vi "Read.vi"(2 "Que name":string, 5 "error in":errorcluster, 7 "Timeout (default 2s)":i32=2000) -> (4 "Message out":string, 6 "error out":errorcluster, 8 "Data":variant)   [LabVIEW 2014, in "Que lib.lvlib"]
uses:
  Que lib.lvlib
  Controls/Queue cluster.ctl
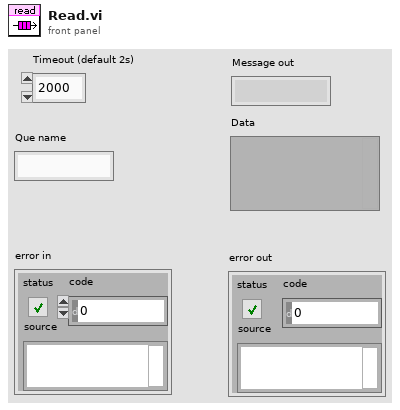
[diagram p1: front panel]
types:
  T1 = typedef "Que lib.lvlib/Queue cluster.ctl" = cluster{"Message":string, "Data":variant}
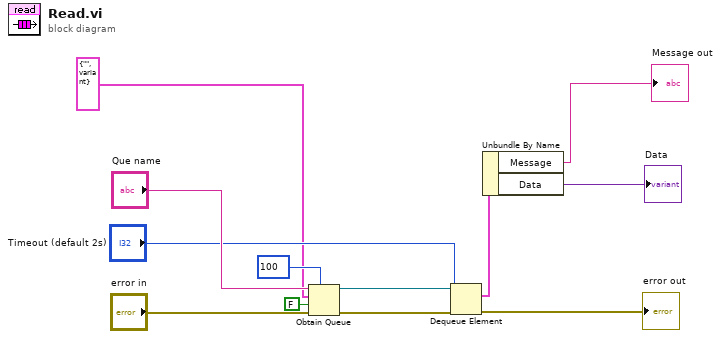
[diagram p0: block diagram]
diagram:
  n1 = Obtain Queue(max queue size (-1, unlimited)=100, name (unnamed)="Que name", element data type=T1 {"Message"="", "Data"=variant} ("Queue Cluster"), create if not found? (T)=FALSE, error in (no error)="error in") -> (queue out=w7:refnum<queue>, error out=w12:errorcluster)  [unwired: 1 out]
  n2 = Dequeue Element(queue=w7, timeout in ms (-1)="Timeout (default 2s)", error in (no error)=w12) -> (element=w3:T1, error out=→"error out":errorcluster)  [unwired: 2 out]
  n3 = Unbundle By Name(w3) -> ("Message"=→"Message out":string, "Data"=→"Data":variant)
